vi "图像处理.vi"(0 "imaq creat":T1, 1 "Image Src":T1, 2 "边缘检测":T1, 3 "Number of Classes":i32=4, 4 "滤波":T1, 5 "error in (no error)":errorcluster, 6 "3D view":T1, 7 "United":T1) -> (12 "overlay":T1, 13 "Ellipse":T2 {"Minor Axis"."Point 2"."Y" format="%.2f"; "Minor Axis"."Point 2"."X" format="%.2f"; "Minor Axis"."Point 1"."Y" format="%.2f"; "Minor Axis"."Point 1"."X" format="%.2f"; "Major Axis"."Point 2"."Y" format="%.2f"; "Major Axis"."Point 2"."X" format="%.2f"; "Major Axis"."Point 1"."Y" format="%.2f"; "Major Axis"."Point 1"."X" format="%.2f"; "Center"."Y" format="%.2f"; "Center"."X" format="%.2f"}, 14 "3D":T1, 15 "灰度图像":T1, 16 "Measurements":cluster{"Area":dbl, "Perimeter":dbl} {"Perimeter" format="%.2f"; "Area" format="%.2f"}, 17 "Centroid":cluster{"X Centroid":sgl, "Y Centroid":sgl} {"Y Centroid" format="%.2f"; "X Centroid" format="%.2f"}, 19 "error out":errorcluster)   [LabVIEW 2015]
uses:
  <vilib>/vision/Image Controls.llb/IMAQ Image.ctl
  <vilib>/vision/NI_Vision_Development_Module.lvlib
panel:
  out "element 4":dbl
  out "element 3":dbl
  out "element 2":dbl
  out "element":dbl
  in  "Real-World Measurements (Particle Analysis 1)":i32[](array[ring]) items=["Center of Mass X", "Center of Mass Y", "First Pixel X", "First Pixel Y", "Bounding Rect Left", "Bounding Rect Top", "Bounding Rect Right", "Bounding Rect Bottom", "Max Feret Diameter Start X", "Max Feret Diameter Start Y", "Max Feret Diameter End X", "Max Feret Diameter End Y", "Max Horiz. Segment Length Left", "Max Horiz. Segment Length Right", "Max Horiz. Segment Length Row", "-", "Bounding Rect Width", "Bounding Rect Height", "Bounding Rect Diagonal", "Perimeter", "Convex Hull Perimeter", "Holes' Perimeter", "Max Feret Diameter", "Equivalent Ellipse Major Axis", "Equivalent Ellipse Minor Axis", "Equivalent Ellipse Minor Axis (Feret)", "Equivalent Rect Long Side", "Equivalent Rect Short Side", "Equivalent Rect Diagonal", "Equivalent Rect Short Side (Feret)", "Average Horiz. Segment Length", "Average Vert. Segment Length", "Hydraulic Radius", "Waddel Disk Diameter", "-", "Area", "Holes' Area", "Particle & Holes' Area", "Convex Hull Area", "Image Area", "-", "Number of Holes", "Number of Horiz. Segments", "Number of Vert. Segments", "-", "Orientation", "Max Feret Diameter Orientation", "-", "% Area/Image Area", "% Area/(Particle & Holes' Area)", "Ratio of Equivalent Ellipse Axes", "Ratio of Equivalent Rect Sides", "-", "Elongation Factor", "Compactness Factor", "Heywood Circularity Factor", "Type Factor", "-", "Sum X", "Sum Y", "Sum XX", "Sum XY", "Sum YY", "Sum XXX", "Sum XXY", "Sum XYY", "Sum YYY", "-", "Moment of Inertia XX", "Moment of Inertia XY", "Moment of Inertia YY", "Moment of Inertia XXX", "Moment of Inertia XXY", "Moment of Inertia XYY", "Moment of Inertia YYY", "Norm. Moment of Inertia XX", "Norm. Moment of Inertia XY", "Norm. Moment of Inertia YY", "Norm. Moment of Inertia XXX", "Norm. Moment of Inertia XXY", "Norm. Moment of Inertia XYY", "Norm. Moment of Inertia YYY", "Hu Moment 1", "Hu Moment 2", "Hu Moment 3", "Hu Moment 4", "Hu Moment 5", "Hu Moment 6", "Hu Moment 7"]
  in  "Pixel Measurements (Particle Analysis 1)":i32[](array[ring])=[0, 1, 2, 3, 4, 5, 6, 7, 41, 42, 43] items=["Center of Mass X", "Center of Mass Y", "First Pixel X", "First Pixel Y", "Bounding Rect Left", "Bounding Rect Top", "Bounding Rect Right", "Bounding Rect Bottom", "Max Feret Diameter Start X", "Max Feret Diameter Start Y", "Max Feret Diameter End X", "Max Feret Diameter End Y", "Max Horiz. Segment Length Left", "Max Horiz. Segment Length Right", "Max Horiz. Segment Length Row", "-", "Bounding Rect Width", "Bounding Rect Height", "Bounding Rect Diagonal", "Perimeter", "Convex Hull Perimeter", "Holes' Perimeter", "Max Feret Diameter", "Equivalent Ellipse Major Axis", "Equivalent Ellipse Minor Axis", "Equivalent Ellipse Minor Axis (Feret)", "Equivalent Rect Long Side", "Equivalent Rect Short Side", "Equivalent Rect Diagonal", "Equivalent Rect Short Side (Feret)", "Average Horiz. Segment Length", "Average Vert. Segment Length", "Hydraulic Radius", "Waddel Disk Diameter", "-", "Area", "Holes' Area", "Particle & Holes' Area", "Convex Hull Area", "Image Area", "-", "Number of Holes", "Number of Horiz. Segments", "Number of Vert. Segments", "-", "Orientation", "Max Feret Diameter Orientation", "-", "% Area/Image Area", "% Area/(Particle & Holes' Area)", "Ratio of Equivalent Ellipse Axes", "Ratio of Equivalent Rect Sides", "-", "Elongation Factor", "Compactness Factor", "Heywood Circularity Factor", "Type Factor", "-", "Sum X", "Sum Y", "Sum XX", "Sum XY", "Sum YY", "Sum XXX", "Sum XXY", "Sum XYY", "Sum YYY", "-", "Moment of Inertia XX", "Moment of Inertia XY", "Moment of Inertia YY", "Moment of Inertia XXX", "Moment of Inertia XXY", "Moment of Inertia XYY", "Moment of Inertia YYY", "Norm. Moment of Inertia XX", "Norm. Moment of Inertia XY", "Norm. Moment of Inertia YY", "Norm. Moment of Inertia XXX", "Norm. Moment of Inertia XXY", "Norm. Moment of Inertia XYY", "Norm. Moment of Inertia YYY", "Hu Moment 1", "Hu Moment 2", "Hu Moment 3", "Hu Moment 4", "Hu Moment 5", "Hu Moment 6", "Hu Moment 7"]
  in  "Connectivity 4/8 (8) (Particle Analysis 1)":bool=TRUE
  out "Particle Measurements (Real-World) (Particle Analysis 1)":dbl[][](array[numeric]) format="%.2f"
  out "Particle Measurements (Pixels) (Particle Analysis 1)":dbl[][](array[numeric]) format="%.2f"
  out "Number of Particles (Particle Analysis 1)":i32
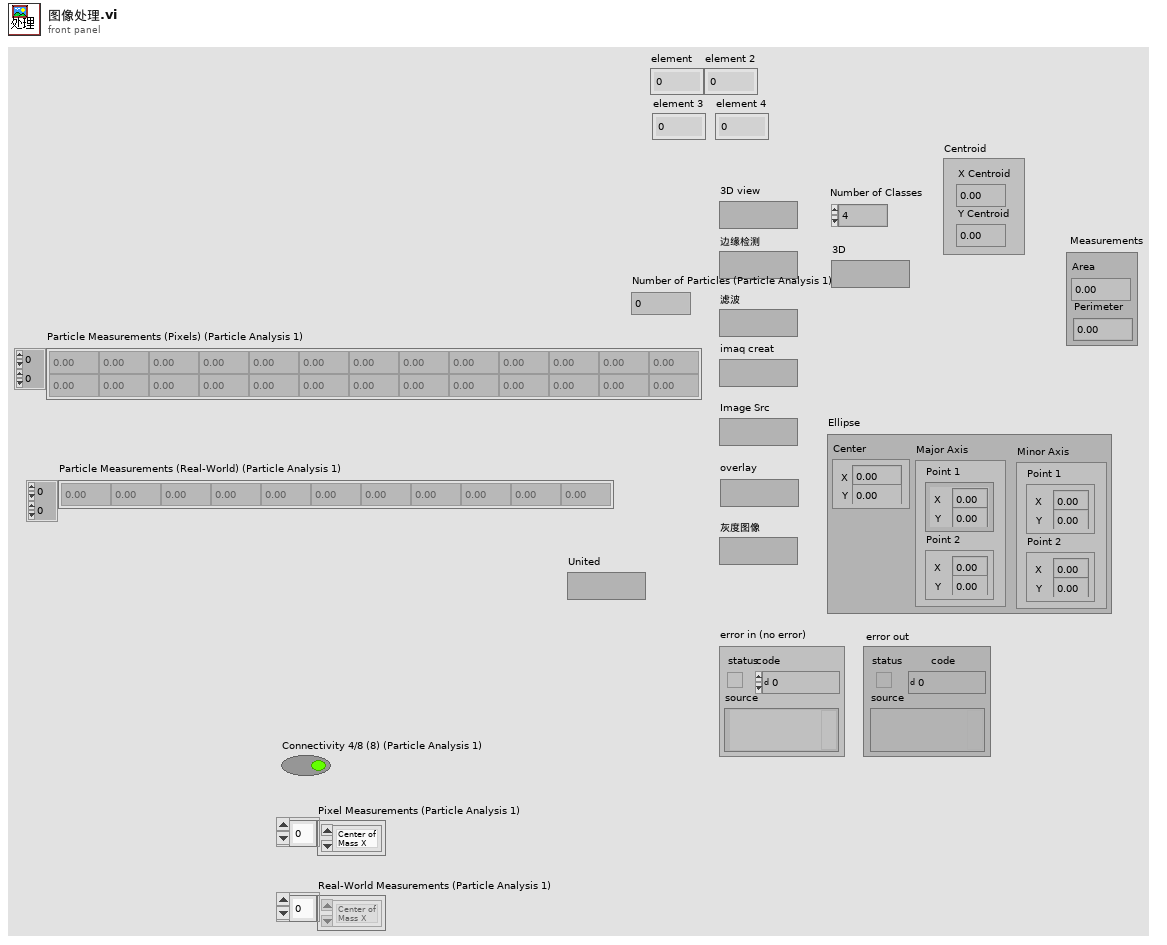
[diagram p1: front panel]
types:
  T1 = typedef "IMAQ Image.ctl" = refnum<image>
  T2 = cluster{"Center":cluster{"X":sgl, "Y":sgl}, "Major Axis":cluster{"Point 1":cluster{"X":sgl, "Y":sgl}, "Point 2":cluster{"X":sgl, "Y":sgl}}, "Minor Axis":cluster{"Point 1":cluster{"X":sgl, "Y":sgl}, "Point 2":cluster{"X":sgl, "Y":sgl}}}
  T3 = enum32{"Differentiation", "Gradient", "Prewitt", "Roberts", "Sigma", "Sobel"}
  T4 = cluster{"Lower value":sgl, "Upper value":sgl, "Replace Value":sgl, "Keep/Replace Value (Replace)":bool}[]
  T5 = cluster{"Lower value":sgl, "Upper value":sgl, "Replace Value":sgl, "Keep/Replace Value (Replace)":bool}
  T6 = cluster{"Numeric":dbl, "Numeric":dbl, "Numeric":dbl, "Numeric":dbl, "element":dbl}
  T7 = typedef "ROI Descriptor" = cluster{"Global Rectangle":i32[], "Contours":cluster{"ID":enum32{"External", "Internal"}, "Type":u32, "Coordinates":i32[]}[]}
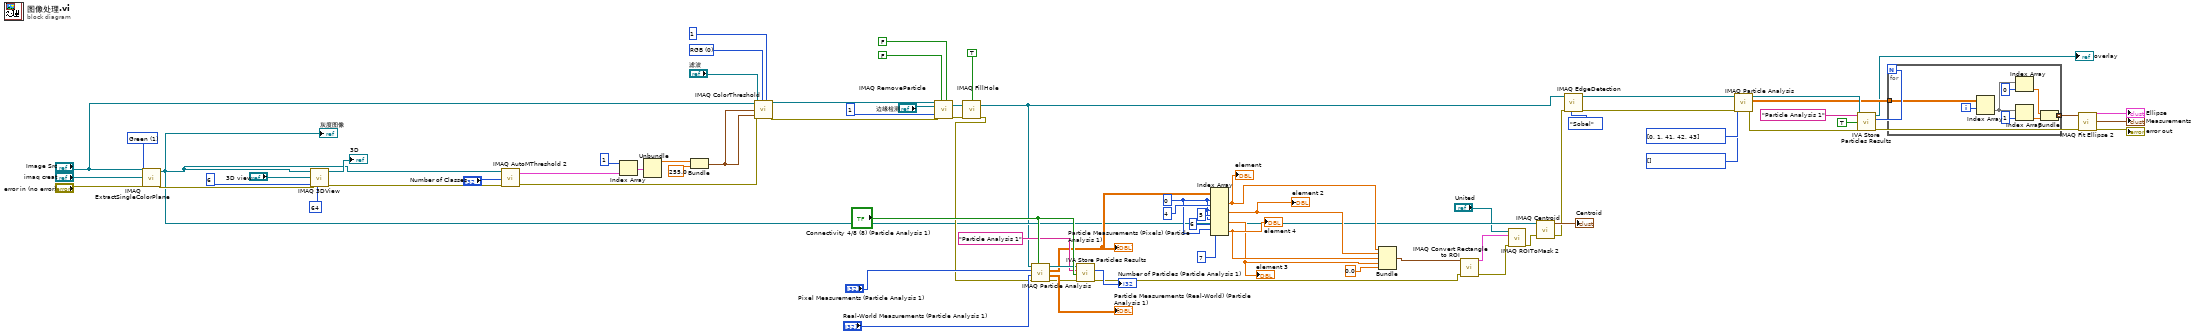
[diagram p0: block diagram]
diagram:
  w20 = 0 ("index (row)")
  w43 = 1 items=["Red", "Green", "Blue", "Hue", "Saturation", "Luminance", "Value", "Intensity"] ("Color Plane")
  w49 = i32[] [] items=["Center of Mass X", "Center of Mass Y", "First Pixel X", "First Pixel Y", "Bounding Rect Left", "Bounding Rect Top", "Bounding Rect Right", "Bounding Rect Bottom", "Max Feret Diameter Start X", "Max Feret Diameter Start Y", "Max Feret Diameter End X", "Max Feret Diameter End Y", "Max Horiz. Segment Length Left", "Max Horiz. Segment Length Right", "Max Horiz. Segment Length Row", "-", "Bounding Rect Width", "Bounding Rect Height", "Bounding Rect Diagonal", "Perimeter", "Convex Hull Perimeter", "Holes' Perimeter", "Max Feret Diameter", "Equivalent Ellipse Major Axis", "Equivalent Ellipse Minor Axis", "Equivalent Ellipse Minor Axis (Feret)", "Equivalent Rect Long Side", "Equivalent Rect Short Side", "Equivalent Rect Diagonal", "Equivalent Rect Short Side (Feret)", "Average Horiz. Segment Length", "Average Vert. Segment Length", "Hydraulic Radius", "Waddel Disk Diameter", "-", "Area", "Holes' Area", "Particle & Holes' Area", "Convex Hull Area", "Image Area", "-", "Number of Holes", "Number of Horiz. Segments", "Number of Vert. Segments", "-", "Orientation", "Max Feret Diameter Orientation", "-", "% Area/Image Area", "% Area/(Particle & Holes' Area)", "Ratio of Equivalent Ellipse Axes", "Ratio of Equivalent Rect Sides", "-", "Elongation Factor", "Compactness Factor", "Heywood Circularity Factor", "Type Factor", "-", "Sum X", "Sum Y", "Sum XX", "Sum XY", "Sum YY", "Sum XXX", "Sum XXY", "Sum XYY", "Sum YYY", "-", "Moment of Inertia XX", "Moment of Inertia XY", "Moment of Inertia YY", "Moment of Inertia XXX", "Moment of Inertia XXY", "Moment of Inertia XYY", "Moment of Inertia YYY", "Norm. Moment of Inertia XX", "Norm. Moment of Inertia XY", "Norm. Moment of Inertia YY", "Norm. Moment of Inertia XXX", "Norm. Moment of Inertia XXY", "Norm. Moment of Inertia XYY", "Norm. Moment of Inertia YYY", "Hu Moment 1", "Hu Moment 2", "Hu Moment 3", "Hu Moment 4", "Hu Moment 5", "Hu Moment 6", "Hu Moment 7"] ("Real-World Measurements")
  w50 = i32[] [0, 1, 41, 42, 43] items=["Center of Mass X", "Center of Mass Y", "First Pixel X", "First Pixel Y", "Bounding Rect Left", "Bounding Rect Top", "Bounding Rect Right", "Bounding Rect Bottom", "Max Feret Diameter Start X", "Max Feret Diameter Start Y", "Max Feret Diameter End X", "Max Feret Diameter End Y", "Max Horiz. Segment Length Left", "Max Horiz. Segment Length Right", "Max Horiz. Segment Length Row", "-", "Bounding Rect Width", "Bounding Rect Height", "Bounding Rect Diagonal", "Perimeter", "Convex Hull Perimeter", "Holes' Perimeter", "Max Feret Diameter", "Equivalent Ellipse Major Axis", "Equivalent Ellipse Minor Axis", "Equivalent Ellipse Minor Axis (Feret)", "Equivalent Rect Long Side", "Equivalent Rect Short Side", "Equivalent Rect Diagonal", "Equivalent Rect Short Side (Feret)", "Average Horiz. Segment Length", "Average Vert. Segment Length", "Hydraulic Radius", "Waddel Disk Diameter", "-", "Area", "Holes' Area", "Particle & Holes' Area", "Convex Hull Area", "Image Area", "-", "Number of Holes", "Number of Horiz. Segments", "Number of Vert. Segments", "-", "Orientation", "Max Feret Diameter Orientation", "-", "% Area/Image Area", "% Area/(Particle & Holes' Area)", "Ratio of Equivalent Ellipse Axes", "Ratio of Equivalent Rect Sides", "-", "Elongation Factor", "Compactness Factor", "Heywood Circularity Factor", "Type Factor", "-", "Sum X", "Sum Y", "Sum XX", "Sum XY", "Sum YY", "Sum XXX", "Sum XXY", "Sum XYY", "Sum YYY", "-", "Moment of Inertia XX", "Moment of Inertia XY", "Moment of Inertia YY", "Moment of Inertia XXX", "Moment of Inertia XXY", "Moment of Inertia XYY", "Moment of Inertia YYY", "Norm. Moment of Inertia XX", "Norm. Moment of Inertia XY", "Norm. Moment of Inertia YY", "Norm. Moment of Inertia XXX", "Norm. Moment of Inertia XXY", "Norm. Moment of Inertia XYY", "Norm. Moment of Inertia YYY", "Hu Moment 1", "Hu Moment 2", "Hu Moment 3", "Hu Moment 4", "Hu Moment 5", "Hu Moment 6", "Hu Moment 7"] ("Pixel Measurements")
  w75 = u16 0 items=["RGB", "HSL", "HSV", "HSI"] ("Color Mode")
  n1 = call "IMAQ ExtractSingleColorPlane"("Color Plane"=w43, "error in (no error)"="error in (no error)", "Image Dst"="imaq creat", "Image Src"="Image Src") -> ("error out"=w62:errorcluster, "Image Dst Out"=w8:T1)  [unwired: 6 in]
  "灰度图像" <- w8
  n2 = call "IMAQ 3DView"("Maximum height"=64, "error in (no error)"=w62, "Size reduction"=6, "Image Dst"="3D view", "Image Src"=w8) -> ("error out"=w61:errorcluster, "Image Dst Out"=→"3D":T1)  [unwired: 5 in]
  n3 = call "IMAQ AutoMThreshold 2"("error in (no error)"=w61, "Number of Classes"="Number of Classes", "Image"=w8) -> ("error out"=w68:errorcluster, "Threshold Data out"=w74:T4)  [unwired: 1 in, 1 out]
  n4 = Index Array(array=w74, index=1) -> (element=w72:T5)
  n5 = Unbundle(w72) -> ("Lower value"=w71:sgl)  [unwired: 3 out]
  n6 = Bundle("Lower value"=w71, 255.0) -> (w69:cluster{"Lower value":sgl, dbl})  [unwired: 1 in]
  n7 = call "IMAQ ColorThreshold"("Blue or Luma or Val or Inten Range"=w69, "Replace Value"=1, "Green or Sat Range"=w69, "Color Mode"=w75, "error in (no error)"=w68, "Red or Hue Range"=w69, "Image Dst"="滤波", "Image Src"="Image Src") -> ("error out"=w51:errorcluster, "Image Dst Out"=w53:T1)  [unwired: 2 out]
  n8 = call "IMAQ RemoveParticle"("Connectivity 4/8 (8)"=FALSE, "Square/Hexa (Square)"=FALSE, "error in (no error)"=w51, "Number of Erosion"=1, "Image Dst"="边缘检测", "Image Src"=w53) -> ("error out"=w58:errorcluster, "Image Dst Out"=w56:T1)  [unwired: 1 in, 3 out]
  n9 = call "IMAQ FillHole"("error in (no error)"=w58, "Image Src"=w56, "Connectivity 4/8 (8)"=TRUE) -> ("error out"=w25:errorcluster, "Image Dst Out"=w4:T1)  [unwired: 1 in, 2 out]
  n10 = call "IMAQ Particle Analysis"("Connectivity 4/8 (8)"="Connectivity 4/8 (8) (Particle Analysis 1)", "error in (no error)"=w25, "Real-World Measurements"="Real-World Measurements (Particle Analysis 1)", "Pixel Measurements"="Pixel Measurements (Particle Analysis 1)", "Image"=w4) -> ("error out"=w27:errorcluster, "Particle Measurements (Real-World)"=→"Particle Measurements (Real-World) (Particle Analysis 1)":dbl[][], "Particle Measurements (Pixels)"=w24:dbl[][], "Image Out (duplicate)"=w29:T1)  [unwired: 3 out]
  "Particle Measurements (Pixels) (Particle Analysis 1)" <- w24
  n11 = call <vilib>:"IVA Store Particles Results.vi"("error in (no error)"=w27, "Connectivity 4/8 (8)"="Connectivity 4/8 (8) (Particle Analysis 1)", "Step Name"="Particle Analysis 1", "Image in"=w29) -> ("error out"=w11:errorcluster, "Number of Particles"=→"Number of Particles (Particle Analysis 1)":i32)  [unwired: 6 out]
  n12 = Index Array(array=w24, index (row) #1=w20, index (col) #1=4 ("disabled index (col)"), index (row) #2=w20, index (col) #2=5 ("disabled index (col)"), index (row) #3=w20, index (col) #3=6 ("disabled index (col)"), index (row) #4=w20, index (col) #4=7 ("disabled index (col)")) -> (element #1=w17:dbl, element #2=w16:dbl, element #3=w14:dbl, element #4=w15:dbl)
  "element" <- w17
  "element 2" <- w16
  "element 3" <- w14
  "element 4" <- w15
  n13 = Bundle("Numeric"=w17, "Numeric"=w16, "Numeric"=w15, "Numeric"=w14, "element"=0.0) -> (w12:T6)  [unwired: 1 in]
  n14 = call "IMAQ Convert Rectangle to ROI"("error in (no error)"=w11, "Rectangle"=w12) -> ("error out"=w10:errorcluster, "ROI Descriptor"=w18:T7)  [unwired: 7 in]
  n15 = call "IMAQ ROIToMask 2"("error in (no error)"=w10, "ROI Descriptor"=w18, "Image"="United") -> ("error out"=w9:errorcluster)  [unwired: 6 in, 2 out]
  n16 = call "IMAQ Centroid"("error in (no error)"=w9, "Image"=w8) -> ("error out"=w3:errorcluster, "Centroid"=→"Centroid":cluster{"X Centroid":sgl, "Y Centroid":sgl})  [unwired: 2 in]
  n17 = call "IMAQ EdgeDetection"("Method"=T3."Sobel", "error in (no error)"=w3, "Image Src"=w4) -> ("error out"=w2:errorcluster, "Image Dst Out"=w1:T1)  [unwired: 3 in, 4 out]
  n18 = call "IMAQ Particle Analysis"("error in (no error)"=w2, "Real-World Measurements"=w49, "Pixel Measurements"=w50, "Image"=w1) -> ("error out"=w46:errorcluster, "Particle Measurements (Pixels)"=w47:dbl[][], "Image Out (duplicate)"=w48:T1)  [unwired: 1 in, 4 out]
  n19 = call <vilib>:"IVA Store Particles Results.vi"("error in (no error)"=w46, "Connectivity 4/8 (8)"=TRUE, "Step Name"="Particle Analysis 1", "Image in"=w48) -> ("error out"=w64:errorcluster, "Number of Particles"=w66:i32, "Image dup"=→"overlay":T1)  [unwired: 5 out]
  n20 = for {
    N: w66 -> [_]
    tunnel: w47 -> [w82]
    tunnel: [w83] -> w65 mode=indexing
    i -> [w81]
    n21 = Index Array(array=w82, index (row)=w81) -> (element=w80:dbl[])  [unwired: 1 in]
    n22 = Index Array(array=w80, index=0) -> (element=w79:dbl)
    n23 = Index Array(array=w80, index=1) -> (element=w78:dbl)
    n24 = Bundle("Numeric"=w79, "Numeric"=w78) -> (w83:cluster{"Numeric":dbl, "Numeric":dbl})  [unwired: 1 in]
  }
  n25 = call "IMAQ Fit Ellipse 2"("error in (no error)"=w64, "Radial Points"=w65) -> ("error out"=→"error out":errorcluster, "Measurements"=→"Measurements":cluster{"Area":dbl, "Perimeter":dbl}, "Ellipse"=→"Ellipse":T2)  [unwired: 4 in, 3 out]
